vi "KMeans.vi"(8 "error in":errorcluster) -> (0 "error out":errorcluster, 3 "out":refnum<class "KMeans.lvclass">)   [LabVIEW 2020]
doc: "K-Means clustering.\n\n Read more in the :ref:`User Guide <k_means>`.\n\n Parameters\n ----------\n\n n_clusters : int, default=8\n The number of clusters to form as well as the number of\n centroids to generate.\n\n init : {'k-means++', 'random'}, callable or array-like of shape (n_clusters, n_features), default='k-means++'\n Method for initialization:\n\n 'k-means++' : selects initial cluster centers for k-mean\n clustering in a smart way to speed up convergence. See section\n Notes in k_init for more details.\n\n 'random': choose `n_clusters` observations (rows) at random from data\n for the initial centroids.\n\n If an array is passed, it should be of shape (n_clusters, n_features)\n and gives the initial centers.\n\n If a callable is passed, it should take arguments X, n_clusters and a\n random state and return an initialization.\n\n n_init : int, default=10\n Number of time the k-means algorithm will be run with different\n centroid seeds. The final results will be the best output of\n n_init consecutive runs in terms of inertia.\n\n max_iter : int, default=300\n Maximum number of iterations of the k-means algorithm for a\n single run.\n\n tol : float, default=1e-4\n Relative tolerance with regards to Frobenius norm of the difference\n in the cluster centers of two consecutive iterations to declare\n convergence.\n\n precompute_distances : {'auto', True, False}, default='auto'\n Precompute distances (faster but takes more memory).\n\n 'auto' : do not precompute distances if n_samples * n_clusters > 12\n million. This corresponds to about 100MB overhead per job using\n double precision.\n\n True : always precompute distances.\n\n False : never precompute distances.\n\n .. deprecated:: 0.23\n 'precompute_distances' was deprecated in version 0.22 and will be\n removed in 1.0 (renaming of 0.25). It has no effect.\n\n verbose : int, default=0\n Verbosity mode.\n\n random_state : int, RandomState instance or None, default=None\n Determines random number generation for centroid initialization. Use\n an int to make the randomness deterministic.\n See :term:`Glossary <random_state>`.\n\n copy_x : bool, default=True\n When pre-computing distances it is more numerically accurate to center\n the data first. If copy_x is True (default), then the original data is\n not modified. If False, the original data is modified, and put back\n before the function returns, but small numerical differences may be\n introduced by subtracting and then adding the data mean. Note that if\n the original data is not C-contiguous, a copy will be made even if\n copy_x is False. If the original data is sparse, but not in CSR format,\n a copy will be made even if copy_x is False.\n\n n_jobs : int, default=None\n The number of OpenMP threads to use for the computation. Parallelism is\n sample-wise on the main cython loop which assigns each sample to its\n closest center.\n\n ``None`` or ``-1`` means using all processors.\n\n .. deprecated:: 0.23\n ``n_jobs`` was deprecated in version 0.23 and will be removed in\n 1.0 (renaming of 0.25).\n\n algorithm : {\"auto\", \"full\", \"elkan\"}, default=\"auto\"\n K-means algorithm to use. The classical EM-style algorithm is \"full\".\n The \"elkan\" variation is more efficient on data with well-defined\n clusters, by using the triangle inequality. However it's more memory\n intensive due to the allocation of an extra array of shape\n (n_samples, n_clusters).\n\n For now \"auto\" (kept for backward compatibiliy) chooses \"elkan\" but it\n might change in the future for a better heuristic.\n\n .. versionchanged:: 0.18\n Added Elkan algorithm\n\n Attributes\n ----------\n cluster_centers_ : ndarray of shape (n_clusters, n_features)\n Coordinates of cluster centers. If the algorithm stops before fully\n converging (see ``tol`` and ``max_iter``), these will not be\n consistent with ``labels_``.\n\n labels_ : ndarray of shape (n_samples,)\n Labels of each point\n\n inertia_ : float\n Sum of squared distances of samples to their closest cluster center.\n\n n_iter_ : int\n Number of iterations run.\n\n See Also\n --------\n MiniBatchKMeans : Alternative online implementation that does incremental\n updates of the centers positions using mini-batches.\n For large scale learning (say n_samples > 10k) MiniBatchKMeans is\n probably much faster than the default batch implementation.\n\n Notes\n -----\n The k-means problem is solved using either Lloyd's or Elkan's algorithm.\n\n The average complexity is given by O(k n T), where n is the number of\n samples and T is the number of iteration.\n\n The worst case complexity is given by O(n^(k+2/p)) with\n n = n_samples, p = n_features. (D. Arthur and S. Vassilvitskii,\n 'How slow is the k-means method?' SoCG2006)\n\n In practice, the k-means algorithm is very fast (one of the fastest\n clustering algorithms available), but it falls in local minima. That's why\n it can be useful to restart it several times.\n\n If the algorithm stops before fully converging (because of ``tol`` or\n ``max_iter``), ``labels_`` and ``cluster_centers_`` will not be consistent,\n i.e. the ``cluster_centers_`` will not be the means of the points in each\n cluster. Also, the estimator will reassign ``labels_`` after the last\n iteration to make ``labels_`` consistent with ``predict`` on the training\n set.\n\n \nAvailable methods:\nGet Attributes\nGet Params\nSet Params"
uses:
  KMeans.lvclass
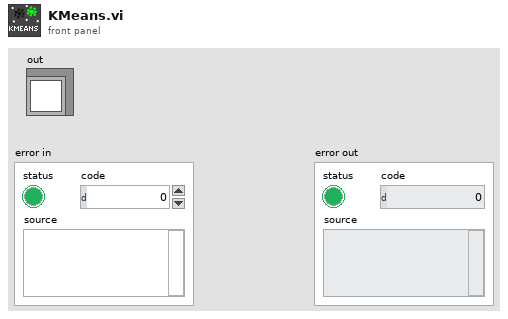
[diagram p1: front panel]
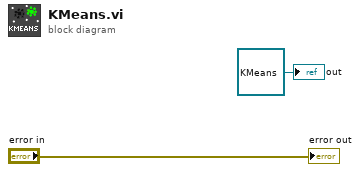
[diagram p0: block diagram]
diagram:
  "out" <- refnum<class "KMeans.lvclass"> refnum ("model")
  "error out" <- "error in"
